vi "Picture Probe.vi"(1 "Picture In":picture) -> (0 "Pause if TRUE":bool)   [LabVIEW 2017]
doc: "Displays the picture and includes the Height and Width of the image."
panel:
  out "Height:":i16
  out "Picture":picture
  out "Width:":i16
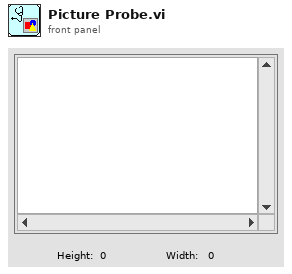
[diagram p1: front panel]
types:
  T1 = typedef "imagedata.ctl" = cluster{"image type":i32, "image depth":i32, "image":u8[], "mask":u8[], "colors":u32[], "Rectangle":cluster{"left":i16, "top":i16, "right":i16, "bottom":i16}}
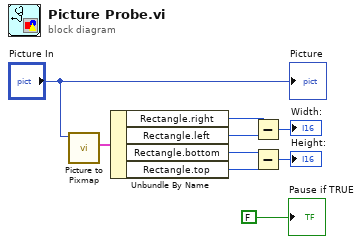
[diagram p0: block diagram]
diagram:
  n1 = call <vilib>:"Picture to Pixmap.vi"("picture"="Picture In") -> ("image data"=w1:T1)  [unwired: 9 in, 1 out]
  n2 = Unbundle By Name(w1) -> ("Rectangle.right"=w8:i16, "Rectangle.left"=w7:i16, "Rectangle.bottom"=w5:i16, "Rectangle.top"=w4:i16)
  n3 = Subtract(x=w8, y=w7) -> (x-y=→"Width:":i16)
  n4 = Subtract(x=w5, y=w4) -> (x-y=→"Height:":i16)
  "Pause if TRUE" <- FALSE
  "Picture" <- "Picture In"
